vi "Concatenate Msg Strings.vi"(11 "StringsIn":string[](array[string])) -> (3 "StringsOut":string[](array[string]))   [LabVIEW 2012]
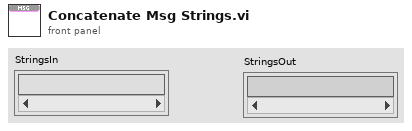
[diagram p1: front panel]
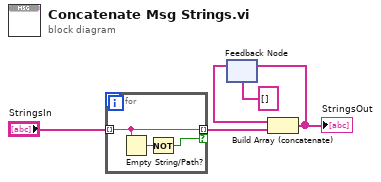
[diagram p0: block diagram]
diagram:
  n1 = for {
    tunnel: "StringsIn" -> [w8] mode=indexing
    tunnel: [w8] -> w4 mode=indexing if=w6
    n2 = Empty String/Path?(string/path=w8) -> (empty?=w7:bool)
    n3 = Not(x=w7) -> (.not. x?=w6:bool)
  }
  n4 = feedback #1(string[] []) -> (w2:string[])
  n5 = Build Array (concatenate)(w2, w4) -> (w3:string[])
  "StringsOut" <- w3
  n6 = feedback-in #1(w3) -> ()
